vi "Step K2450 Volt.vi"(1 "Action":T4=enum."Identify", 2 "Parameters":variant) -> (6 "Output":variant, 7 "Stop":bool)   [LabVIEW 2020]
doc: "This VI reads a single reading from a Keithley 2001 multimeter. The stop boolean is always false. If no reading is obtained a single zero is returned.\nScott Hannahs, NHMFL-FSU, Nov 1993"
uses:
  Sub Controls/Instrument Actions.ctl
  Sub Controls/Instrument Match.ctl
  Sub Controls/Public.ctl
  Sub Controls/Factory Reset.ctl
  Sub Controls/Scan Output.ctl
  Sub Controls/Instrument IDN.ctl
  Sub Controls/User Event Command.ctl
panel:
  in  "Factory Reset":T1
  out "Start Value":dbl=20.0
  in  "# Steps":u32=20
  in  "# Data Points at step":u32=1
  in  "Index":i32
  in  "Wait After Setting":dbl=5.0 format="%<%M:%S>t"
  out "Time":dbl=1200.0 format="%<%H:%M:%S>t"
  in  "End Value":dbl=20.0
  in  "Step Size":dbl=1.0
  out "Title":string
  in  "Public":T2
  in  "Address":u16(ring)
  out "Model":string
  in  "Instruments":T3[](array[typedef])=[{"Model"="MODEL 2450", "Manufacturer"="KEITHLEY INSTRUMENTS", "Term Character"="", "Wait Time (mS)"=0, "Wait for SRQ"=FALSE, "Type"="Voltage Source Step"}]
  out "Measurement":dbl[](array[numeric]) format="%^_7e"
  in  "VISA resource name":refnum<visa-resource-name>
  # "Term Char"
  # "Wait Time (mS)"
  # "Wait for SRQ?"
  # "Type"
  # "Manufacturer"
  # "Model"
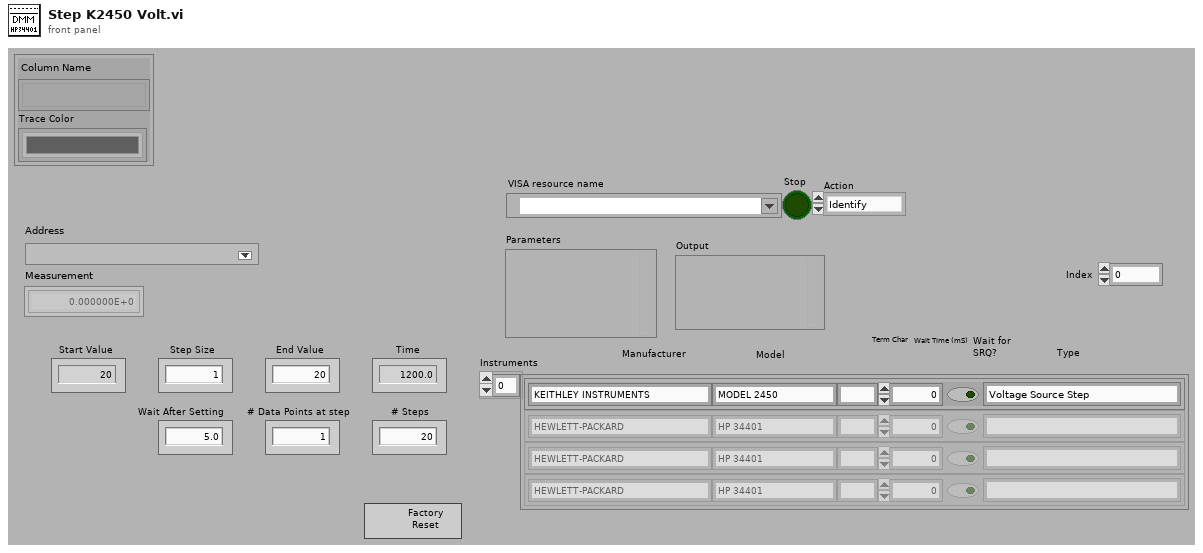
[diagram p1: front panel]
types:
  T1 = typedef "Factory Reset.ctl" = bool
  T2 = typedef "Public.ctl" = cluster{"Column Name":string[], "Trace Color":u32[]}
  T3 = typedef "Instrument Match.ctl" = cluster{"Model":string, "Manufacturer":string, "Term Character":string, "Wait Time (mS)":u32, "Wait for SRQ":bool, "Type":string}
  T4 = typedef "Instrument Actions.ctl" = enum16{"Scan", "Identify", "New", "Configure", "Initialize", "Test", "Read", "Close"}
  T5 = typedef "Scan Output.ctl" = cluster{"Manufacturer":string, "Model":string, "Info":string, "Revision":string, "error out":errorcluster}
  T6 = typedef "Instrument IDN.ctl" = cluster{"VISA Address":string, "Status":u16, "Manufacturer":string, "Model":string, "Info":string, "Info 2":string, "Misc Data":variant}
  T7 = typedef "User Event Command.ctl" = enum32{"Stop Config"}
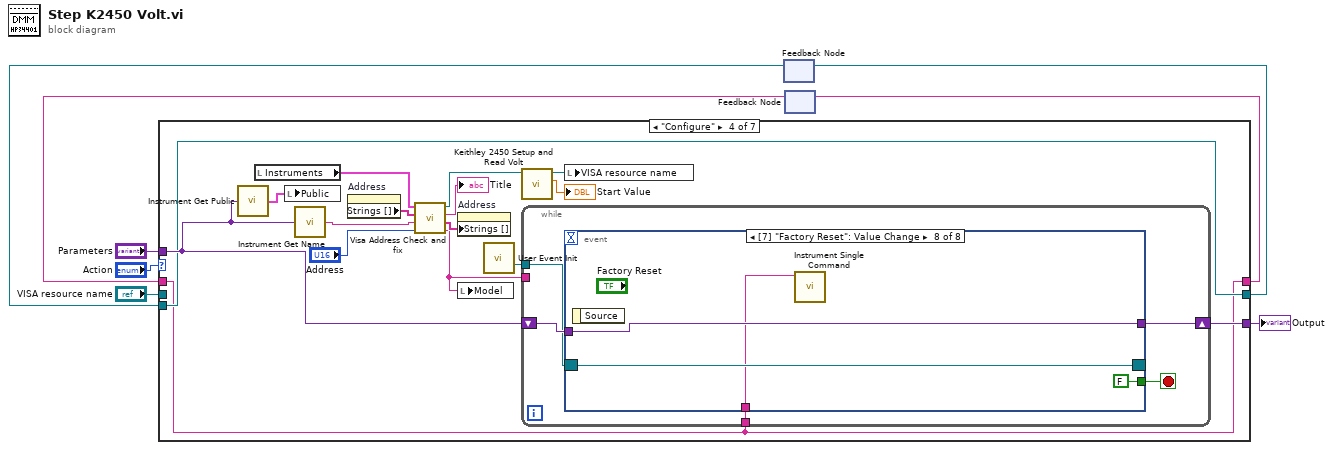
[diagram p0: block diagram]
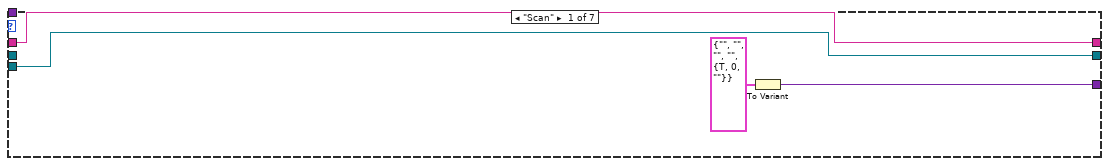
[diagram p2: hidden frame]
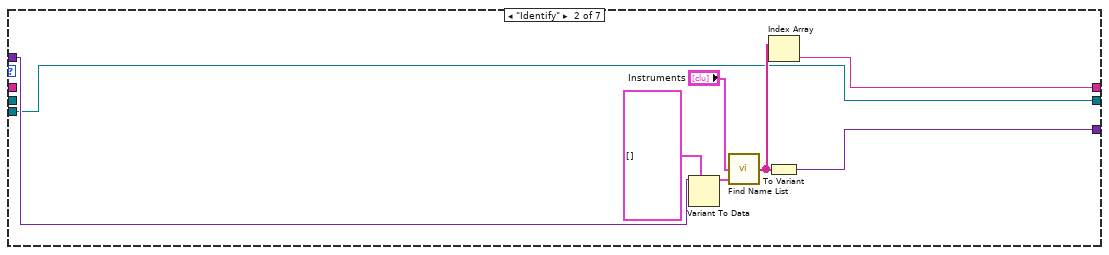
[diagram p3: hidden frame]
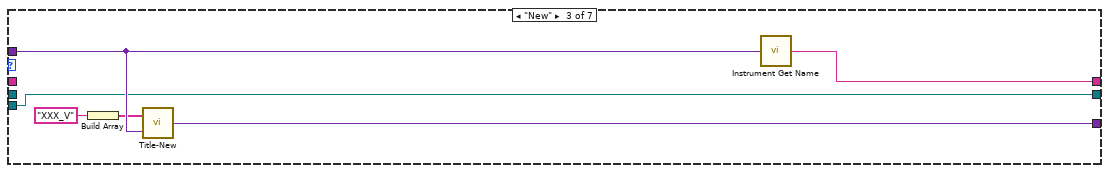
[diagram p4: hidden frame]
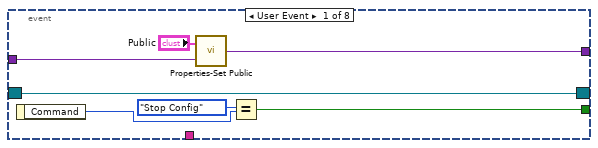
[diagram p5: hidden frame]
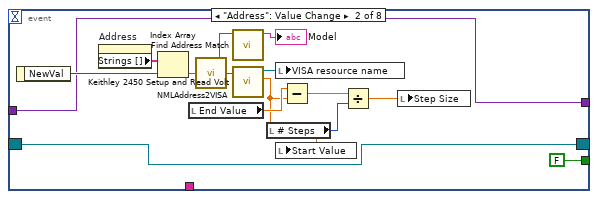
[diagram p6: hidden frame]
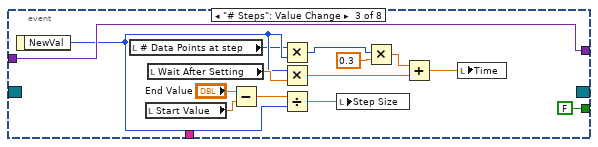
[diagram p7: hidden frame]
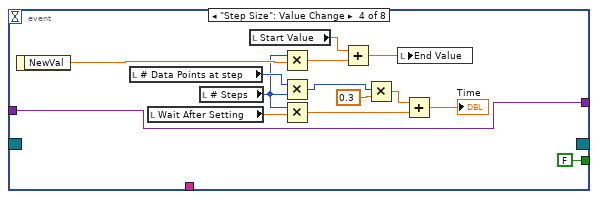
[diagram p8: hidden frame]
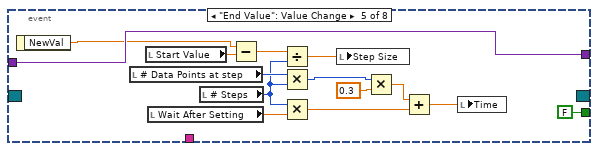
[diagram p9: hidden frame]
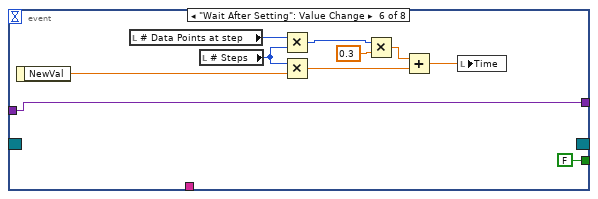
[diagram p10: hidden frame]
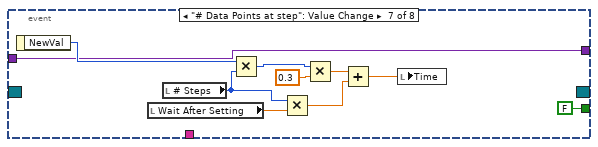
[diagram p11: hidden frame]
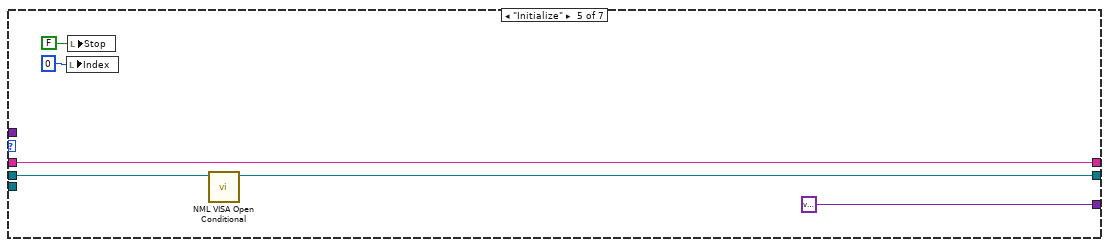
[diagram p12: hidden frame]
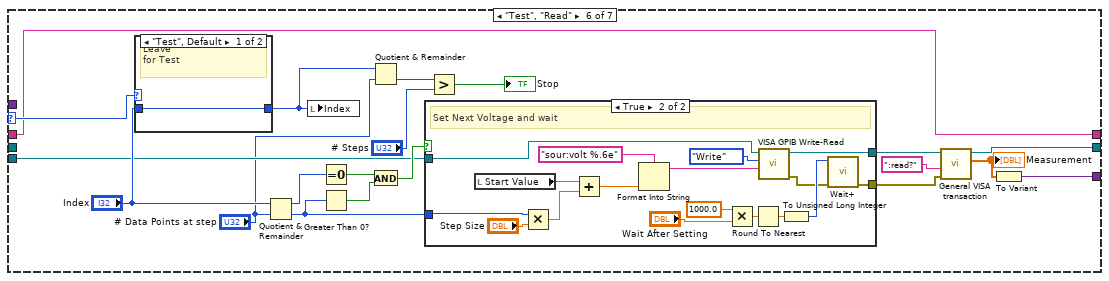
[diagram p13: hidden frame]
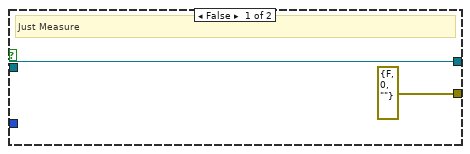
[diagram p14: hidden frame]
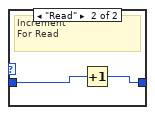
[diagram p15: hidden frame]
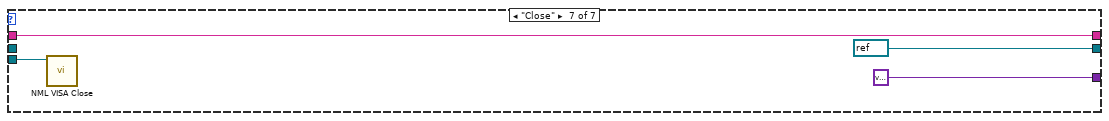
[diagram p16: hidden frame]
diagram:
  n1 = feedback #1() -> (w1:refnum<visa-resource-name>)  [unwired: 1 in]
  n2 = feedback #2() -> (w4:string)  [unwired: 1 in]
  n3 = case shown="\"Configure\"" "Action" {
    selector: "Action" -> [_ _ _ _ _ w158 _]
    tunnel: [w12 w20 w26 w36 variant ("Variant") w160 variant ("Variant")] -> w7
    tunnel: "VISA resource name" -> [_ _ _ _ w140 _ _]
    tunnel: [w11 w15 w23 w27 w138 w157 w185] -> w5
    tunnel: w4 -> [w11 _ _ w27 w138 w157 w185]
    tunnel: "Parameters" -> [_ w19 w25 w34 _ _ _]
    tunnel: [w9 w13 w21 w28 w137 w159 refnum<visa-resource-name> refnum ("Open VISA Resource name")] -> w2
    tunnel: w1 -> [w9 w13 w21 w28 _ w150 w183]
    frame "Scan" {
      n4 = To Variant(anything=T5 {"Manufacturer"="", "Model"="", "Info"="", "Revision"="", "error out"={"status"=TRUE, "code"=0, "source"=""}} ("Scan Output")) -> (Variant=w12:variant)
    }
    frame "Identify" {
      n5 = Variant To Data(type=T6[] [], Variant=w19) -> (data=w17:T6[])  [unwired: 1 in, 1 out]
      n6 = call "Find Name List.vi"("Bus Scan"=w17, "Instruments"="Instruments") -> ("Names"=w14:string[])  [unwired: 1 in]
      n7 = Index Array(array=w14) -> (element=w15:string)  [unwired: 1 in]
      n8 = To Variant(anything=w14) -> (Variant=w20:variant)
    }
    frame "New" {
      n9 = Build Array("XXX_V") -> (w24:string[])
      n10 = call "Title-New.vi"("Parameters"=w25, "Array"=w24) -> ("Instrument Prop"=w26:variant)
      n11 = call "Instrument Get Name.vi"("Parameters"=w25) -> ("Type"=w23:string)
    }
    frame "Configure" {
      n12 = call "Instrument Get Public.vi"("Variant"=w34) -> ("Public"=w37:T2)
      n13 = local read "Instruments"() -> (w39:T3[])
      n14 = local write "Public"(w37) -> ()
      n15 = call "Instrument Get Name.vi"("Parameters"=w34) -> ("Type"=w33:string)
      n16 = property on="Address" class="Ring (strict)"() -> ("Strings []"=w40:string[])  [unwired: 2 in, 2 out]
      n17 = call "Visa Address Check and fix.vi"("Address"="Address", "Name"=w33, "NML Addresses"=w40, "Instruments"=w39) -> ("Model"=w38:string, "NML Addresses"=w42:string[], "Title"=→"Title":string, "VISA resource name"=w31:refnum<visa-resource-name>)  [unwired: 2 out]
      n18 = property on="Address" class="Ring (strict)"("Strings []"=w42) -> ()  [unwired: 2 in, 2 out]
      n19 = local write "Model"(w38) -> ()
      n20 = call "User Event Init.vi"() -> ("Event Registration Refnum"=w35:refnum<event-registration>)  [unwired: 14 in, 1 out]
      n21 = call "Keithley 2450 Setup and Read Volt.vi"("VISA Refnum in"=w31) -> ("Voltage"=→"Start Value":dbl, "VISA Refnum out"=w30:refnum<visa-resource-name>)  [unwired: 8 in, 1 out]
      n22 = while {
        tunnel: w38 -> [_]
        tunnel: w35 -> [w44]
        shift-right: [w47] -> w36
        shift-left: w34 -> [w45]
        tunnel: w27 -> [w43]
        stop <- w46 stop-if-true
        n23 = event shown="[7] \"Factory Reset\": Value Change" {
          selector: w44 -> [w48 w62 _ _ _ _ _ w133]
          dyn-events: [w48 w62 _ _ _ _ _ w133] -> _
          timeout: _ -> [_ _ _ _ _ _ _ _]
          tunnel: [w52 w63 w82 w96 w110 w112 w122 w134] -> w47
          tunnel: [w50 FALSE FALSE FALSE FALSE FALSE FALSE FALSE] -> w46
          tunnel: w45 -> [w53 w63 w82 w96 w110 w112 w122 w134]
          tunnel: w43 -> [_ _ _ _ _ _ _ w131]
          event User Event {
            n24 = event-data() -> ("Command"=w54:T7)  [unwired: 1 in]
            n25 = call "Properties-Set Public.vi"("Variant"=w53, "New Public"="Public") -> ("Variant 2"=w52:variant)
            n26 = Equal?(x=User_Event_Command."Stop Config", y=w54) -> (x = y?=w50:bool)
          }
          event "Address": Value Change {
            n27 = event-data() -> ("NewVal"=w68:u16)  [unwired: 1 in]
            n28 = property on="Address" class="Ring (strict)"() -> ("Strings []"=w65:string[])  [unwired: 2 in, 2 out]
            n29 = Index Array(array=w65, index=w68) -> (element=w66:string)
            n30 = local read "End Value"() -> (w59:dbl)
            n31 = call "NMLAddress2VISA.vi"("NML Address"=w66) -> ("VISA resource name"=w61:refnum<visa-resource-name>)
            n32 = call "Find Address Match.vi"("VISA resource name"=w61) -> ("Model"=→"Model":string)  [unwired: 3 in, 3 out]
            n33 = call "Keithley 2450 Setup and Read Volt.vi"("VISA Refnum in"=w61) -> ("Voltage"=w56:dbl, "VISA Refnum out"=w60:refnum<visa-resource-name>)  [unwired: 8 in, 1 out]
            n34 = local read "# Steps"() -> (w55:u32)
            n35 = local write "VISA resource name"(w60) -> ()
            n36 = local write "Start Value"(w56) -> ()
            n37 = Subtract(x=w59, y=w56) -> (x-y=w58:dbl)
            n38 = Divide(x=w58, y=w55) -> (x/y=w57:dbl)
            n39 = local write "Step Size"(w57) -> ()
          }
          event "# Steps": Value Change {
            n40 = event-data() -> ("NewVal"=w77:u32)  [unwired: 1 in]
            n41 = local read "# Data Points at step"() -> (w76:u32)
            n42 = local read "Start Value"() -> (w81:dbl)
            n43 = local read "Wait After Setting"() -> (w78:dbl)
            n44 = Subtract(x="End Value", y=w81) -> (x-y=w80:dbl)
            n45 = Multiply(x=w76, y=w77) -> (x*y=w75:u32)
            n46 = Multiply(x=w77, y=w78) -> (x*y=w72:dbl)
            n47 = Divide(x=w80, y=w77) -> (x/y=w79:dbl)
            n48 = local write "Step Size"(w79) -> ()
            n49 = Multiply(x=w75, y=0.3) -> (x*y=w73:dbl)
            n50 = Add(x=w73, y=w72) -> (x+y=w71:dbl)
            n51 = local write "Time"(w71) -> ()
          }
          event "Step Size": Value Change {
            n52 = event-data() -> ("NewVal"=w93:dbl)  [unwired: 1 in]
            n53 = local read "# Data Points at step"() -> (w92:u32)
            n54 = local read "Wait After Setting"() -> (w94:dbl)
            n55 = local read "# Steps"() -> (w85:u32)
            n56 = local read "Start Value"() -> (w86:dbl)
            n57 = Multiply(x=w85, y=w93) -> (x*y=w95:dbl)
            n58 = Multiply(x=w92, y=w85) -> (x*y=w91:u32)
            n59 = Multiply(x=w85, y=w94) -> (x*y=w88:dbl)
            n60 = Add(x=w86, y=w95) -> (x+y=w87:dbl)
            n61 = Multiply(x=w91, y=0.3) -> (x*y=w89:dbl)
            n62 = local write "End Value"(w87) -> ()
            n63 = Add(x=w89, y=w88) -> (x+y=→"Time":dbl)
          }
          event "End Value": Value Change {
            n64 = event-data() -> ("NewVal"=w99:dbl)  [unwired: 1 in]
            n65 = local read "# Data Points at step"() -> (w105:u32)
            n66 = local read "Start Value"() -> (w109:dbl)
            n67 = local read "Wait After Setting"() -> (w106:dbl)
            n68 = local read "# Steps"() -> (w98:u32)
            n69 = Subtract(x=w99, y=w109) -> (x-y=w108:dbl)
            n70 = Divide(x=w108, y=w98) -> (x/y=w107:dbl)
            n71 = Multiply(x=w105, y=w98) -> (x*y=w104:u32)
            n72 = Multiply(x=w98, y=w106) -> (x*y=w101:dbl)
            n73 = local write "Step Size"(w107) -> ()
            n74 = Multiply(x=w104, y=0.3) -> (x*y=w102:dbl)
            n75 = Add(x=w102, y=w101) -> (x+y=w100:dbl)
            n76 = local write "Time"(w100) -> ()
          }
          event "Wait After Setting": Value Change {
            n77 = event-data() -> ("NewVal"=w113:dbl)  [unwired: 1 in]
            n78 = local read "# Data Points at step"() -> (w120:u32)
            n79 = local read "# Steps"() -> (w115:u32)
            n80 = Multiply(x=w120, y=w115) -> (x*y=w119:u32)
            n81 = Multiply(x=w115, y=w113) -> (x*y=w117:dbl)
            n82 = Multiply(x=w119, y=0.3) -> (x*y=w118:dbl)
            n83 = Add(x=w118, y=w117) -> (x+y=w116:dbl)
            n84 = local write "Time"(w116) -> ()
          }
          event "# Data Points at step": Value Change {
            n85 = event-data() -> ("NewVal"=w123:u32)  [unwired: 1 in]
            n86 = local read "Wait After Setting"() -> (w124:dbl)
            n87 = local read "# Steps"() -> (w126:u32)
            n88 = Multiply(x=w123, y=w126) -> (x*y=w130:u32)
            n89 = Multiply(x=w126, y=w124) -> (x*y=w128:dbl)
            n90 = Multiply(x=w130, y=0.3) -> (x*y=w129:dbl)
            n91 = Add(x=w129, y=w128) -> (x+y=w127:dbl)
            n92 = local write "Time"(w127) -> ()
          }
          event Value Change {
            n93 = event-data() -> ()  [unwired: 1 in, 1 out]
            n94 = call "Instrument Single Command.vi"("VISA Name"=w131) -> ()  [unwired: 10 in, 1 out]
          }
        }
      }
      n95 = local write "VISA resource name"(w30) -> ()
    }
    frame "Initialize" {
      n96 = local write "Index"(0 ("Index")) -> ()
      n97 = local write "Stop"(FALSE ("Stop")) -> ()
      n98 = call "NML VISA Open Conditional.vi"("VISA resource name"=w140) -> ("dup VISA Session"=w137:refnum<visa-resource-name>)  [unwired: 8 in, 2 out]
    }
    frame "Test", "Read" {
      n99 = case shown="\"Test\", Default" w158 {
        tunnel: "Index" -> [w180 w182]
        tunnel: [w180 w181] -> w146
        frame "Test", Default {
          # "Leave\nfor Test"
        }
        frame "Read" {
          # "Increment \nFor Read"
          n100 = Increment(x=w182) -> (x+1=w181:i32)
        }
      }
      n101 = Quotient & Remainder(x="Index", y="# Data Points at step") -> (x-y*floor(x/y)=w156:u32, floor(x/y)=w151:u32)
      n102 = local write "Index"(w146) -> ()
      n103 = Equal To 0?(x=w156) -> (x = 0?=w155:bool)
      n104 = Greater Than 0?(x=w151) -> (x > 0?=w154:bool)
      n105 = Quotient & Remainder(x=w146, y="# Data Points at step") -> (floor(x/y)=w144:u32)  [unwired: 1 out]
      n106 = And(x=w155, y=w154) -> (x .and. y?=w153:bool)
      n107 = case shown="True" w153 {
        tunnel: w151 -> [_ w176]
        tunnel: w150 -> [w162 w174]
        tunnel: [w162 w173] -> w149
        tunnel: [errorcluster {"status"=FALSE, "code"=0, "source"=""} ("error out") w164] -> w141
        frame False {
          # "Just Measure"
        }
        frame True {
          # "Set Next Voltage and wait"
          n108 = local read "Start Value"() -> (w179:dbl)
          n109 = Multiply(x=w176, y="Step Size") -> (x*y=w178:dbl)
          n110 = Add(x=w179, y=w178) -> (x+y=w171:dbl)
          n111 = Format Into String(format string="sour:volt %.6e", w171) -> (resulting string=w175:string)  [unwired: 2 in, 1 out]
          n112 = Multiply(x=1000.0, y="Wait After Setting") -> (x*y=w167:dbl)
          n113 = Round To Nearest(number=w167) -> (nearest integer value=w166:dbl)
          n114 = call "VISA GPIB Write-Read.vi"("Command"=w175, "Action"=enum16{"Write", "Read", "Write & Read"}."Write", "VISA resource name"=w174) -> ("error out"=w163:errorcluster, "dup VISA Session"=w173:refnum<visa-resource-name>)  [unwired: 5 in, 2 out]
          n115 = To Unsigned Long Integer(number=w166) -> (unsigned 32bit integer=w169:u32)
          n116 = call "Wait+.vi"("Error In"=w163, "milliseconds to wait"=w169) -> ("Error Out"=w164:errorcluster)  [unwired: 4 in, 1 out]
        }
      }
      n117 = Greater?(x=w144, y="# Steps") -> (0:→"Stop":bool)
      n118 = call "General VISA transaction.vi"("error in (no error)"=w141, "Command String"=":read?", "VISA Session"=w149) -> ("Measurement"=w147:dbl[], "dup VISA Session"=w159:refnum<visa-resource-name>)  [unwired: 3 in, 4 out]
      "Measurement" <- w147
      n119 = To Variant(anything=w147) -> (Variant=w160:variant)
    }
    frame "Close" {
      n120 = call "NML VISA Close.vi"("VISA resource name"=w183) -> ()  [unwired: 10 in, 1 out]
    }
  }
  "Output" <- w7
  n121 = feedback-in #1(w2) -> ()
  n122 = feedback-in #2(w5) -> ()
